vi "stop stuff operes.vi"(9 "reset":bool, 11 "gyro":dbl) -> ()   [LabVIEW 2017]
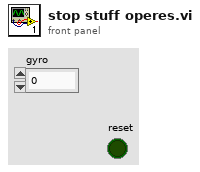
[diagram p1: front panel]
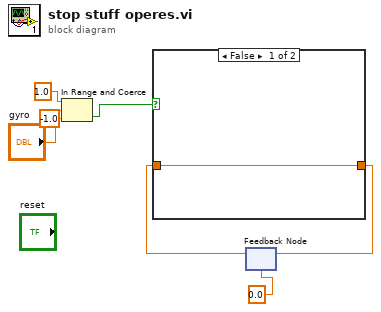
[diagram p0: block diagram]
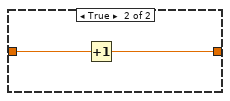
[diagram p2: hidden frame]
diagram:
  n1 = In Range and Coerce(upper limit=1.0 ("lower limit"), x="gyro", lower limit=-1.0) -> (In Range?=w4:bool)  [unwired: 1 out]
  n2 = feedback #1(0.0 ("lower limit")) -> (w1:dbl)
  n3 = case shown="False" w4 {
    tunnel: w1 -> [w8 w10]
    tunnel: [w8 w9] -> w2
    frame False {
    }
    frame True {
      n4 = Increment(x=w10) -> (x+1=w9:dbl)
    }
  }
  n5 = feedback-in #1(w2) -> ()
